vi "CMD_08T_SetSetpoint.vi"(9 "Setpoint, K":dbl=295.0 min=195.0 max=395.0, 11 "VISA resource name":refnum<visa-resource-name>) -> (3 "VISA resource name out":refnum<visa-resource-name>)   [LabVIEW 2017]
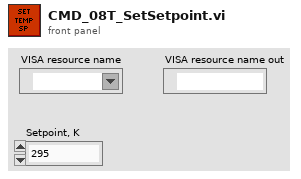
[diagram p1: front panel]
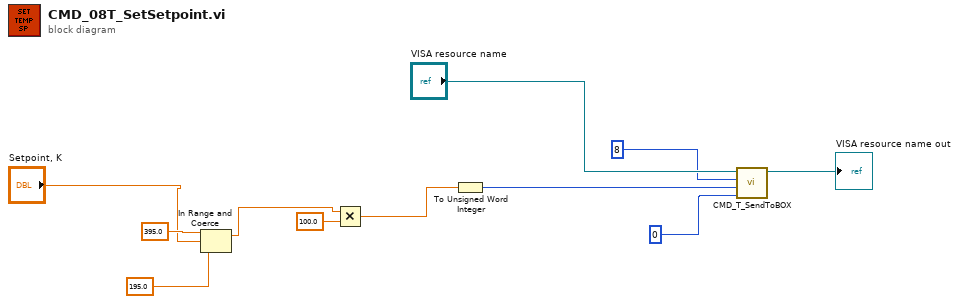
[diagram p0: block diagram]
diagram:
  n1 = In Range and Coerce(upper limit=395.0, x="Setpoint, K", lower limit=195.0) -> (coerced(x)=w1:dbl)  [unwired: 1 out]
  n2 = Multiply(x=w1, y=100.0) -> (x*y=w6:dbl)
  n3 = To Unsigned Word Integer(number=w6) -> (unsigned 16bit integer=w8:u16)
  n4 = call "CMD_T_SendToBOX.vi"("arg2"=i16 0, "arg1"=w8, "CMD"=i8 8, "VISA resource name"="VISA resource name") -> ("VISA resource name out"=→"VISA resource name out":refnum<visa-resource-name>)  [unwired: 7 in]
